vi "Initialise notifiers and events.vi"(8 "error in (no error)":errorcluster, 11 "SubscriptionDetailsParent in":refnum<class "SubscriptionDetailsParent.lvclass">) -> (0 "error out":errorcluster, 3 "SubscriptionDetailsParent out":refnum<class "SubscriptionDetailsParent.lvclass">)   [LabVIEW 2020, in "wamplv.lvlib" / "SubscriptionDetailsParent.lvclass"]
uses:
  SubscriptionDetailsParent.lvclass
  SubscriptionDetailsParent.lvclass/SubscriptionDetailsParent.ctl
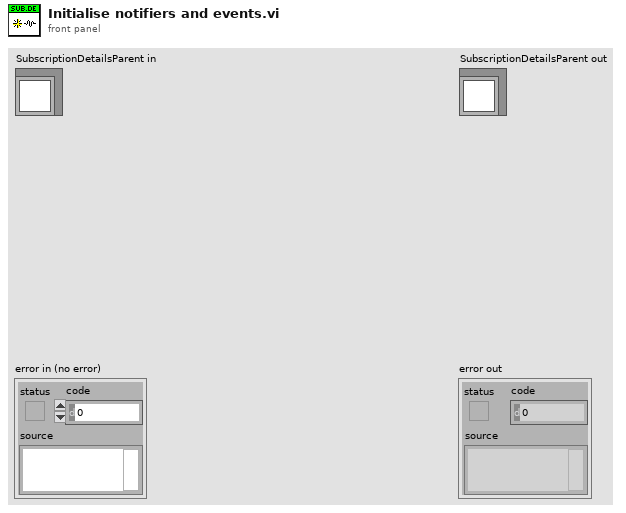
[diagram p1: front panel]
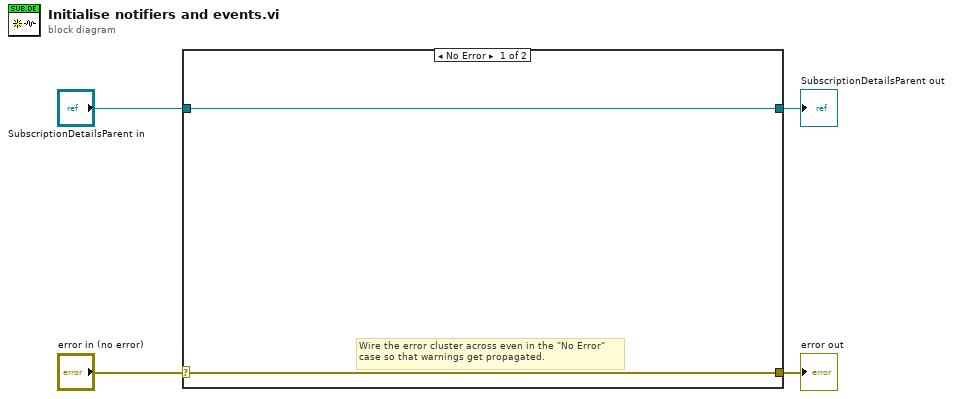
[diagram p0: block diagram]
diagram:
  n1 = case shown="No Error" "error in (no error)" {
    selector: "error in (no error)" -> [w5 w8]
    tunnel: [w5 w8] -> w3
    tunnel: [w6 w7] -> w1
    tunnel: "SubscriptionDetailsParent in" -> [w6 w7]
    frame No Error {
      # "Wire the error cluster across even in the \"No Error\"\ncase so that warnings get propagated."
    }
    frame Error {
    }
  }
  "error out" <- w3
  "SubscriptionDetailsParent out" <- w1
